vi "Channel Name from Enum.vi"(8 "error in (no error)":errorcluster, 10 "Channel Enum":u16=65535, 11 "CIFCorePlugin in":refnum<class "CIFCorePlugin.lvclass">) -> (0 "error out":errorcluster, 2 "Channel Name":string, 3 "CIFCorePlugin out":refnum<class "CIFCorePlugin.lvclass">)   [LabVIEW 2021, in "CIFCorePlugin.lvclass"]
uses:
  CIFCorePlugin.lvclass
  CIFCorePlugin.lvclass/CIFCorePlugin.ctl
  CIFUtilities/CIFChannelMng/CIFChannelMng.lvclass/CIFChannelMng.ctl
  CIFUtilities/CIFClocks/SubVIs/Add Error.vi
  Common/Utilities/Append Error Location.vi
  CIFUtilities/CIFChannelMng/CIFChannelMng.lvclass
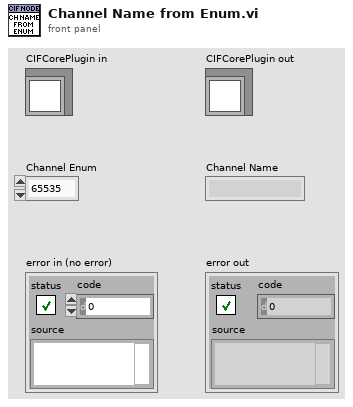
[diagram p1: front panel]
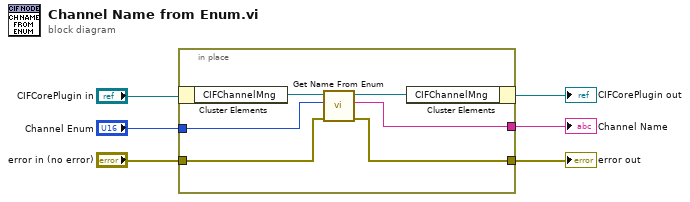
[diagram p0: block diagram]
diagram:
  n1 = in-place {
    in-place-border: "error in (no error)" -> [w10]
    in-place-border: [w9] -> w5
    in-place-border: "Channel Enum" -> [w8]
    in-place-border: [w7] -> w1
    n2 = in-place-cluster #1("CIFCorePlugin in") -> ("CIFChannelMng"=w12:refnum<class "CIFChannelMng.lvclass">)
    n3 = call "Get Name From Enum.vi"("error in (no error)"=w10, "Channel Enum"=w8, "CIFChannelMng in"=w12) -> ("error out"=w9:errorcluster, "Channel Name out"=w7:string, "CIFChannelMng out"=w11:refnum<class "CIFChannelMng.lvclass">)  [unwired: 6 in]
    n4 = in-place-cluster #1("CIFChannelMng"=w11) -> (→"CIFCorePlugin out":refnum<class "CIFCorePlugin.lvclass">)
  }
  "error out" <- w5
  "Channel Name" <- w1
